vi "Bounding Box to Rectangle ROI (LV 2013 SP1)_2.vi"(11 "Bounding Box":cluster{"x":sgl, "y":sgl}[](array[cluster])) -> (0 "Left":i16, 1 "Top":i16, 2 "Right":i16, 3 "Bottom":i16)   [LabVIEW 2014]
doc: "Takes Arrays of Matches and filters the Bounding Box for each match. Then prepares coordinates to match rectangle region to allow creating ROIs"
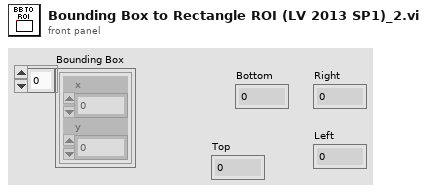
[diagram p1: front panel]
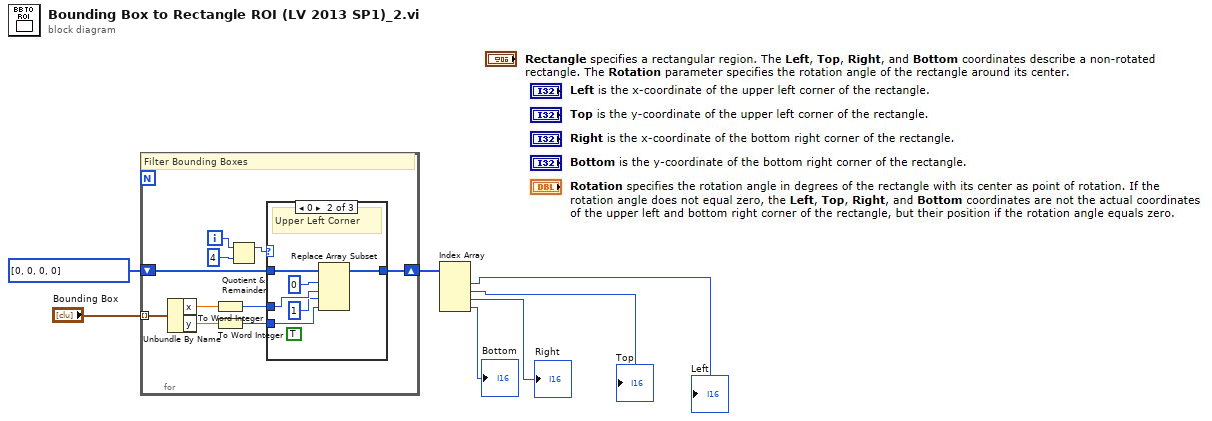
[diagram p0: block diagram]
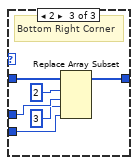
[diagram p3: hidden frame]
diagram:
  n1 = for {
    tunnel: "Bounding Box" -> [w10] mode=indexing
    shift-right: [w8] -> w2
    shift-left: i16[] [0, 0, 0, 0] -> [w9]
    i -> [w16]
    # "Filter Bounding Boxes"
    n2 = Unbundle By Name(w10) -> ("x"=w14:sgl, "y"=w15:sgl)
    n3 = To Word Integer(number=w14) -> (16bit integer=w13:i16)
    n4 = To Word Integer(number=w15) -> (16bit integer=w12:i16)
    n5 = Quotient & Remainder(x=w16, y=4) -> (x-y*floor(x/y)=w11:i32)  [unwired: 1 out]
    n6 = case shown="0" w11 {
      tunnel: w12 -> [_ w20 w26]
      tunnel: w13 -> [_ w22 w28]
      tunnel: w9 -> [w18 w24 w30]
      tunnel: [w18 w19 w25] -> w8
      frame -1, Default {
      }
      frame 0 {
        (unwired) TRUE
        # "Upper Left Corner"
        n7 = Replace Array Subset(array=w24, new element #1=w22, index #1=0, new element #2=w20, index #2=1) -> (w19:i16[])
      }
      frame 2 {
        # "Bottom Right Corner"
        n8 = Replace Array Subset(array=w30, new element #1=w28, index #1=2, new element #2=w26, index #2=3) -> (w25:i16[])
      }
    }
  }
  n9 = Index Array(array=w2) -> (element #1=→"Left":i16, element #2=→"Top":i16, element #3=→"Right":i16, element #4=→"Bottom":i16)  [unwired: 4 in]
